vi "edge_single.vi"(11 "DI Value":bool) -> (3 "DO Value":bool)   [LabVIEW 2017]
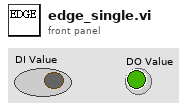
[diagram p1: front panel]
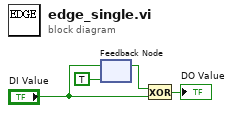
[diagram p0: block diagram]
diagram:
  n1 = feedback #1(TRUE ("DI Value")) -> (w4:bool)
  n2 = feedback-in #1("DI Value") -> ()
  n3 = Exclusive Or(1:"DI Value", 2:w4) -> (0:→"DO Value":bool)
